vi "Sonic Shifter with Single Toggle.vi"   [LabVIEW 2013]
uses:
  Sally_Framework_2014/State_Machine_Enum.ctl
  <vilib>/Rock Robotics/WPI/Solenoid/WPI_SolenoidValue.ctl
  Robot Global Data.vi
  <vilib>/Rock Robotics/WPI/Solenoid/WPI_SolenoidSetEnum.vi
types:
  T1 = typedef "State_Machine_Enum.ctl" = enum16{"Idle", "Start", "Do", "Stop", "Init"}
  T2 = typedef "WPI_SolenoidValue.ctl" = enum16{"Off", "On", "Forward", "Reverse"}
  T3 = typedef "WPI_SolenoidDevRef.ctl" = cluster{"DevStatus":errorcluster, "Solenoid Module":T4, "Forward Solenoid Channel":T5, "Reverse Solenoid Channel":T5}
  T4 = typedef "FPGA_TypedefSolenoidModule.ctl" = enum16{"Solenoid Module 1", "Solenoid Module 2"}
  T5 = typedef "WPI_SolenoidChannel.ctl" = enum8{"Solenoid 1", "Solenoid 2", "Solenoid 3", "Solenoid 4", "Solenoid 5", "Solenoid 6", "Solenoid 7", "Solenoid 8", "Invalid"}
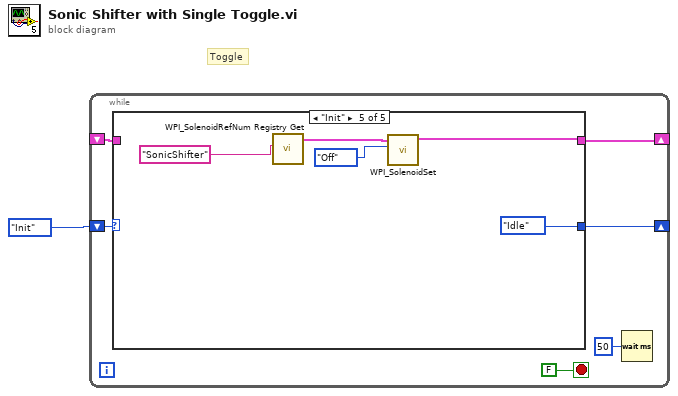
[diagram p0: block diagram]
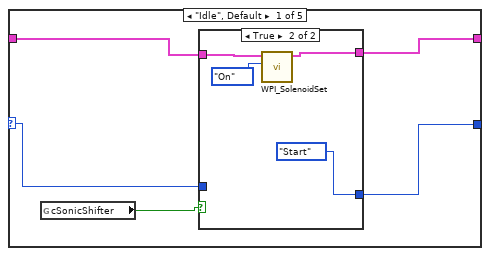
[diagram p2: hidden frame]
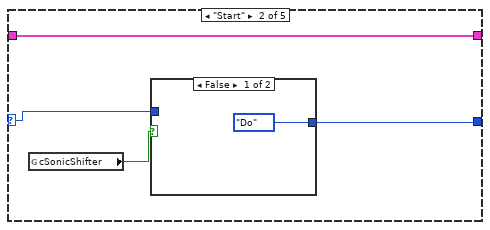
[diagram p4: hidden frame]
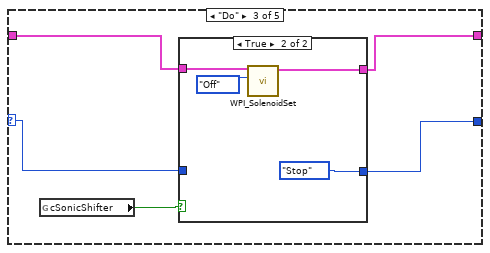
[diagram p6: hidden frame]
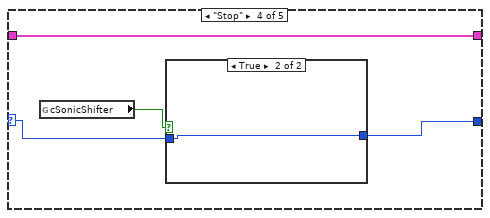
[diagram p8: hidden frame]
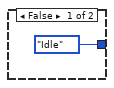
[diagram p9: hidden frame]
diagram:
  # "Toggle"
  n1 = while {
    shift-right: [w6] -> _
    shift-left: State_Machine_Enum."Init" ("State") -> [w7]
    shift-right: [w5] -> _
    shift-left: _ -> [w4]
    stop <- FALSE stop-if-true
    n2 = case shown="\"Init\"" w7 {
      selector: w7 -> [w9 w20 w26 w38 _]
      tunnel: [w10 w21 w27 w39 State_Machine_Enum."Idle" ("State")] -> w6
      tunnel: [w11 w22 w28 w37 w44] -> w5
      tunnel: w4 -> [w12 w22 w29 w37 _]
      frame "Idle", Default {
        n3 = global read "Robot Global Data.vi" "cSonicShifter"() -> (w8:bool)
        n4 = case shown="True" w8 {
          tunnel: w12 -> [w13 w18]
          tunnel: [w13 w17] -> w11
          tunnel: [w14 State_Machine_Enum."Start" ("State")] -> w10
          tunnel: w9 -> [w14 _]
          frame False {
          }
          frame True {
            n5 = call-poly <vilib>:"WPI_SolenoidSet.vi"("Value"=WPI_SolenoidValue."On", "SolenoidDevRef"=w18) -> ("SolenoidDevRef"=w17:T3)  [unwired: 8 in, 1 out]
          }
        }
      }
      frame "Start" {
        n6 = global read "Robot Global Data.vi" "cSonicShifter"() -> (w19:bool)
        n7 = case shown="False" w19 {
          tunnel: [State_Machine_Enum."Do" ("State") w24] -> w21
          tunnel: w20 -> [_ w24]
          frame False {
          }
          frame True {
          }
        }
      }
      frame "Do" {
        n8 = global read "Robot Global Data.vi" "cSonicShifter"() -> (w25:bool)
        n9 = case shown="True" w25 {
          tunnel: w29 -> [w31 w35]
          tunnel: [w31 w34] -> w28
          tunnel: [w30 State_Machine_Enum."Stop" ("State")] -> w27
          tunnel: w26 -> [w30 _]
          frame False {
          }
          frame True {
            n10 = call-poly <vilib>:"WPI_SolenoidSet.vi"("Value"=WPI_SolenoidValue."Off", "SolenoidDevRef"=w35) -> ("SolenoidDevRef"=w34:T3)  [unwired: 8 in, 1 out]
          }
        }
      }
      frame "Stop" {
        n11 = global read "Robot Global Data.vi" "cSonicShifter"() -> (w36:bool)
        n12 = case shown="True" w36 {
          tunnel: [State_Machine_Enum."Idle" ("State") w41] -> w39
          tunnel: w38 -> [_ w41]
          frame False {
          }
          frame True {
          }
        }
      }
      frame "Init" {
        n13 = call <vilib>:"WPI_SolenoidRefNum Registry Get.vi"("refnum name"="SonicShifter") -> ("SolenoidDevRef"=w45:T3)  [unwired: 9 in, 1 out]
        n14 = call-poly <vilib>:"WPI_SolenoidSet.vi"("Value"=WPI_SolenoidValue."Off", "SolenoidDevRef"=w45) -> ("SolenoidDevRef"=w44:T3)  [unwired: 8 in, 1 out]
      }
    }
    n15 = Wait (ms)(milliseconds to wait=u32 50) -> ()  [unwired: 1 out]
  }
